vi "GetFunctionParams.vi"(8 "error in (no error)":errorcluster, 11 "PmuAnalysis in":refnum<class "PmuAnalysis.lvclass">) -> (0 "error out":errorcluster, 2 "FunctionParams":variant, 3 "PmuAnalysis out":refnum<class "PmuAnalysis.lvclass">)   [LabVIEW 2018, in "AnalysisPlugins.lvlib" / "PmuAnalysis.lvclass"]
uses:
  PmuAnalysis.lvclass
  FGen/MemberClasses/PmuTestFunctions/PmuTestFunctions.lvclass
  PmuAnalysis.lvclass/PmuAnalysis.ctl
  FGen/MemberClasses/PmuTestFunctions/PmuTestFunctions.lvclass/PmuTestFunctions.ctl
  Accessors/Read Function.vi
  FGen/MemberClasses/PmuTestFunctions/Accessors/Read PmuTestParams.vi
  FGen/MemberClasses/FunctionBaseClass/FunctionBase.lvclass
panel:
  # "Not all analysis plugins will\nhave function classes"
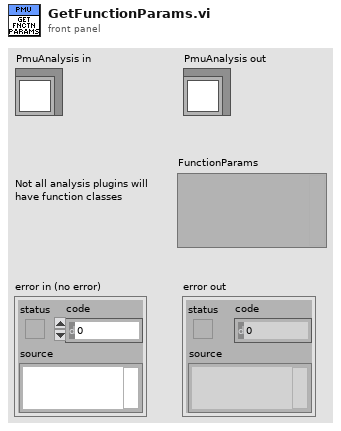
[diagram p1: front panel]
types:
  T1 = typedef "Functions.lvlib/PmuTestFunctions.lvclass/PmuTestParams.ctl" = dbl[][]
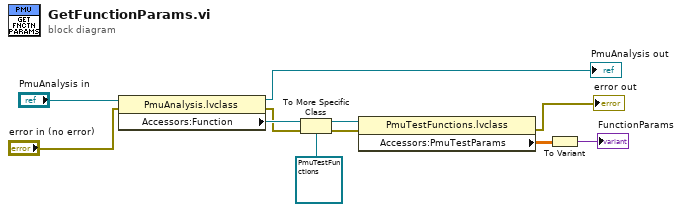
[diagram p0: block diagram]
diagram:
  n1 = property class="PmuAnalysis.lvclass"(reference="PmuAnalysis in", error in="error in (no error)") -> (reference out=→"PmuAnalysis out":refnum<class "PmuAnalysis.lvclass">, error out=w8:errorcluster, "Accessors:Function"=w9:refnum<class "FunctionBase.lvclass">)
  n2 = To More Specific Class(target class=refnum<class "PmuTestFunctions.lvclass"> refnum ("Functions.lvlib:PmuTestFunctions.lvclass"), reference=w9, error in=w8) -> (specific class reference=w5:refnum<class "PmuTestFunctions.lvclass">, error out=w4:errorcluster)
  n3 = property class="PmuTestFunctions.lvclass"(reference=w5, error in=w4) -> (error out=→"error out":errorcluster, "Accessors:PmuTestParams"=w3:T1)  [unwired: 1 out]
  n4 = To Variant(anything=w3) -> (Variant=→"FunctionParams":variant)
